vi "FilterSupportedVirtualChannels.vi"(8 "error in (no error)":errorcluster, 10 "not supported virtual channels":string[](array[string]), 11 "channels in data group":T1[](array[typedef])) -> (0 "error out":errorcluster, 3 "filtered channels in data group":T1[](array[typedef]))   [LabVIEW 2017, in "CmsVirtualChannel.lvlib"]
uses:
  <vilib>/addons/InsightCM/Devices/Shared/Cms/CmsVirtualChannel/CmsVirtualChannel.lvlib
  <vilib>/addons/InsightCM/MessageBus/Base/controls/R2_Channel.ctl
  <vilib>/addons/InsightCM/MessageBus/Base/controls/KeyValuePair.ctl
  <vilib>/addons/InsightCM/MessageBus/Base/controls/Metric.ctl
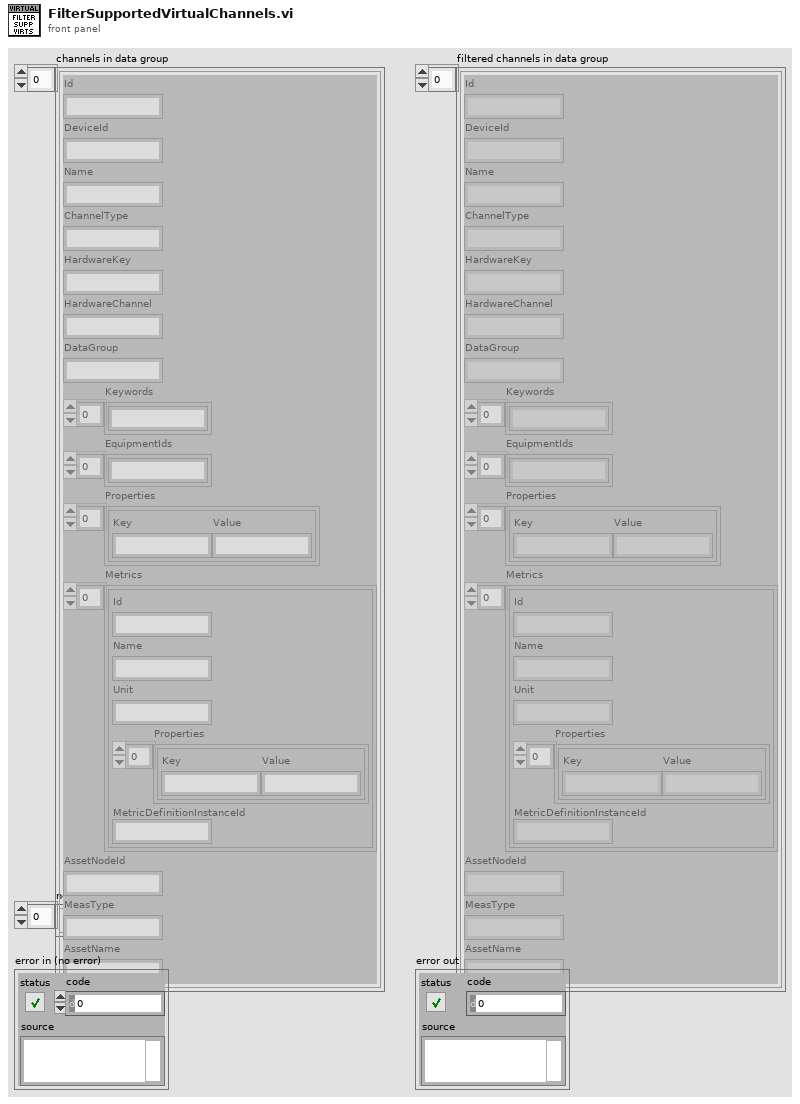
[diagram p1: front panel]
types:
  T1 = typedef "R2_Channel.ctl" = cluster{"Id":string, "DeviceId":string, "Name":string, "ChannelType":string, "HardwareKey":string, "HardwareChannel":string, "DataGroup":string, "Keywords":string[], "EquipmentIds":string[], "Properties":T2[], "Metrics":T3[], "AssetNodeId":string, "MeasType":string, "AssetName":string}
  T2 = typedef "KeyValuePair.ctl" = cluster{"Key":string, "Value":string}
  T3 = typedef "Metric.ctl" = cluster{"Id":string, "Name":string, "Unit":string, "Properties":T2[], "MetricDefinitionInstanceId":string}
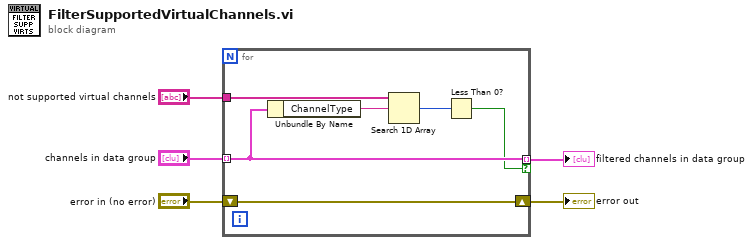
[diagram p0: block diagram]
diagram:
  n1 = for {
    tunnel: "channels in data group" -> [w8] mode=indexing
    shift-right: [w11] -> w3
    shift-left: "error in (no error)" -> [w11]
    tunnel: "not supported virtual channels" -> [w10]
    tunnel: [w8] -> w1 mode=indexing if=w6
    n2 = Unbundle By Name(w8) -> ("ChannelType"=w9:string)
    n3 = Search 1D Array(1D array=w10, element=w9) -> (index of element=w7:i32)  [unwired: 1 in]
    n4 = Less Than 0?(x=w7) -> (x < 0?=w6:bool)
  }
  "filtered channels in data group" <- w1
  "error out" <- w3
